vi "set current selection (single).vi"(8 "error in (no error)":errorcluster, 10 "path":string, 11 "alias-tree in":refnum<class "alias-tree.lvclass">) -> (0 "error out":errorcluster, 1 "invalid path":bool, 3 "alias-tree out":refnum<class "alias-tree.lvclass">)   [LabVIEW 2017, in "vs-tree-utility.lvlib" / "alias-tree.lvclass"]
uses:
  alias-tree.lvclass
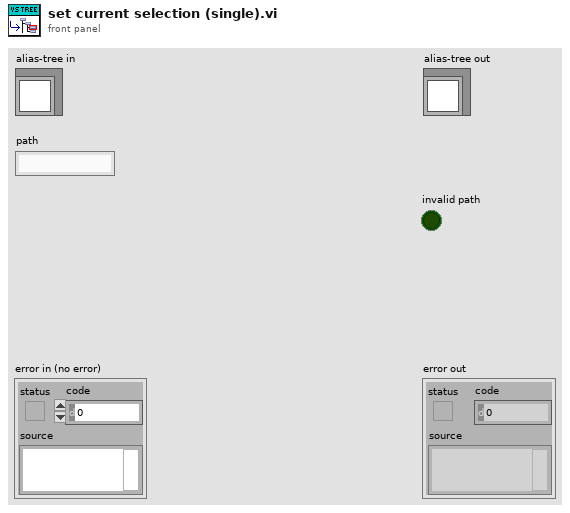
[diagram p1: front panel]
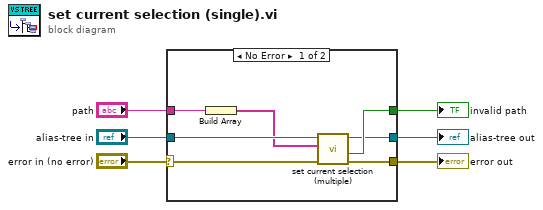
[diagram p0: block diagram]
diagram:
  n1 = case shown="No Error" "error in (no error)" {
    selector: "error in (no error)" -> [w12 w15]
    tunnel: [w8 w15] -> w5
    tunnel: [w7 w14] -> w4
    tunnel: "alias-tree in" -> [w11 w14]
    tunnel: "path" -> [w13 _]
    tunnel: [w9 _] -> w1
    frame No Error {
      n2 = Build Array(w13) -> (w10:string[])
      n3 = call "set current selection (multiple).vi"("error in (no error)"=w12, "paths"=w10, "alias-tree in"=w11) -> ("error out"=w8:errorcluster, "invalid path"=w9:bool, "alias-tree out"=w7:refnum<class "alias-tree.lvclass">)  [unwired: 5 in, 1 out]
    }
    frame Error {
    }
  }
  "error out" <- w5
  "alias-tree out" <- w4
  "invalid path" <- w1
